vi "save_image_no_imaq.vi"(9 "Image index":u32) -> ()   [LabVIEW 2011]
uses:
  <userlib>/atmcd32d.llb/Tiff_type typedef.ctl
  Action Items.ctl
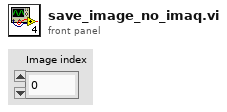
[diagram p1: front panel]
types:
  T1 = typedef "Action Items.ctl" = enum16{"Initialize", "Get"}
  T2 = typedef "Tiff_type typedef.ctl" = enum16{"8-bit", "16-bit", "color"}
  T3 = cluster{"Path":string, "Filestem":string, "Filestem incl time t":string}
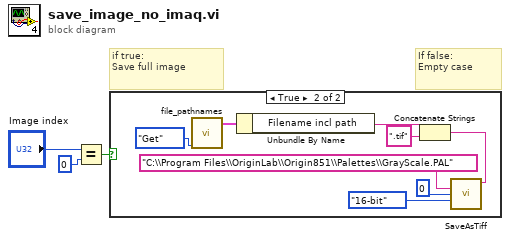
[diagram p0: block diagram]
diagram:
  # "If false:\nEmpty case"
  # "if true: \nSave full image"
  n1 = Equal?(x="Image index", y=u32 0) -> (x = y?=w1:bool)
  n2 = case shown="True" w1 {
    frame False {
    }
    frame True {
      n3 = call "file_pathnames.vi"("Action"=Action_Items."Get") -> ("File-path\n-names"=w8:T3)  [unwired: 10 in]
      n4 = Unbundle By Name(w8) -> ("Filename incl path"=w5:string)
      n5 = Concatenate Strings(w5, ".tif" ("string")) -> (w4:string)
      n6 = call <userlib>:"SaveAsTiff.vi"("path"=w4, "palette"="C:\\Program Files\\OriginLab\\Origin851\\Palettes\\GrayScale.PAL", "position"=0, "type"=Tiff_type_typedef."16-bit") -> ()  [unwired: 10 in, 2 out]
    }
  }
